vi "HVAC Randomize Measurements.vi"(10 "DeviceID":T2) -> (3 "HVAC_Measurement Array out":T1[](array[typedef]))   [LabVIEW 2018, in "IED Test Framework.lvlib" / "IED Test.lvclass"]
uses:
  IED Test.lvclass
  <vilib>/ORNL/CSEISMIC DDS/CSEISMIC DDS Base/Data Types/Controls/DeviceID.ctl
  <vilib>/ORNL/CSEISMIC DDS/CSEISMIC DDS Base/Data Types/HVAC_Measurement.ctl
  <vilib>/ORNL/CSEISMIC DDS/CSEISMIC DDS Base/CSEISMIC DDS.lvclass
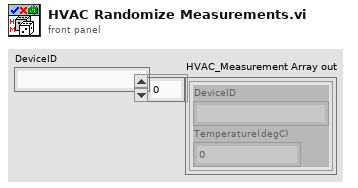
[diagram p1: front panel]
types:
  T1 = typedef "CSEISMIC DDS.lvlib/CSEISMIC DDS.lvclass/HVAC_Measurement.ctl" = cluster{"DeviceID":T2, "Temperature(degC)":dbl}
  T2 = typedef "CSEISMIC DDS.lvlib/CSEISMIC DDS.lvclass/DeviceID.ctl" = string
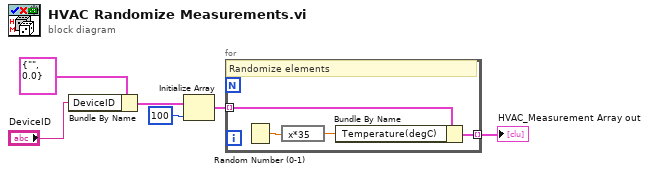
[diagram p0: block diagram]
diagram:
  n1 = Bundle By Name(cluster=T1 {"DeviceID"="", "Temperature(degC)"=0.0} ("HVAC_Measurement"), "DeviceID"="DeviceID") -> (w6:T1)
  n2 = Initialize Array(w6, 100 ("dimension size")) -> (w3:T1[])
  n3 = for {
    tunnel: w3 -> [w10] mode=indexing
    tunnel: [w9] -> w2 mode=indexing
    # "Randomize elements"
    n4 = Random Number (0-1)() -> (number: 0 to 1=w8:dbl)
    n5 = expression code="x*35"(w8) -> (w7:dbl)
    n6 = Bundle By Name(cluster=w10, "Temperature(degC)"=w7) -> (w9:T1)
  }
  "HVAC_Measurement Array out" <- w2
